vi "APC_9049_rpm.vi"(1 "millisecond timer value":u32) -> (0 "rpm from DAQ":dbl)   [LabVIEW 2020]
doc: "This example demonstrates the procedure required to apply different NI-DAQmx Custom Scales to each virtual channel in a task. A DAQmx Task Property Node (Functions >> NI Measurements >> DAQmx - Data Acquisition >> DAQmx Advanced Task Options) is used to obtain the task's virtual channels. A DAQmx Channel Property Node (Functions >> NI Measurements >> DAQmx - Data Acquisition) is then used to set the custom scale for each virtual channel in the task.\n\nThe \"DAQmx Create Scale\" VI creates a custom scale for each channel in the channel list. *Note, make sure your Minimum and Maximum channel parameters are consistent with the range the scale will create."
panel:
  out "Elapsed time":u32
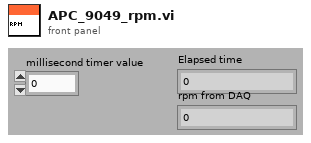
[diagram p1: front panel]
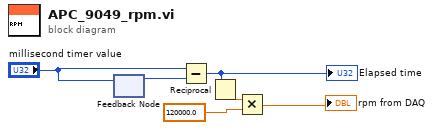
[diagram p0: block diagram]
diagram:
  n1 = feedback #1() -> (w6:u32)  [unwired: 1 in]
  n2 = feedback-in #1("millisecond timer value") -> ()
  n3 = Subtract(x="millisecond timer value", y=w6) -> (x-y=w5:u32)
  "Elapsed time" <- w5
  n4 = Reciprocal(x=w5) -> (1/x=w4:dbl)
  n5 = Multiply(x=w4, y=120000.0) -> (x*y=→"rpm from DAQ":dbl)
